vi "X Table Stage Manufacturer Model - FGV.vi"(7 "Actions":T2=enum."Clear", 8 "Error In":errorcluster, 11 "Device Type [In]":T1 caption="Device Type") -> (0 "Error Out":errorcluster, 3 "X Out":T1 caption="Device Type [Out]")   [LabVIEW 2014]
uses:
  General/Controls/FGV Actions.ctl
  General/Controls/Translation Stage Types.ctl
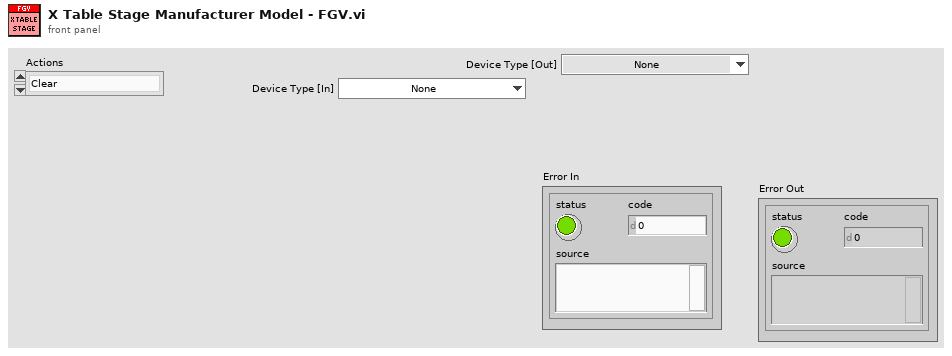
[diagram p1: front panel]
types:
  T1 = typedef "Translation Stage Types.ctl" = enum16{"None", "Thorlabs LTS", "Thorlabs MLJ"}
  T2 = typedef "FGV Actions.ctl" = enum16{"Init", "Set", "Get", "Clear"}
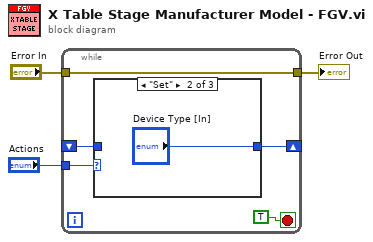
[diagram p0: block diagram]
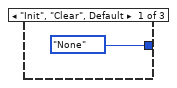
[diagram p2: hidden frame]
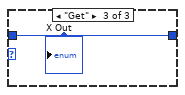
[diagram p3: hidden frame]
diagram:
  n1 = while {
    tunnel: "Actions" -> [w8]
    shift-right: [w6] -> _
    shift-left: _ -> [w5]
    tunnel: [w4] -> w2
    tunnel: "Error In" -> [w4]
    stop <- TRUE stop-if-true
    n2 = case shown="\"Set\"" w8 {
      tunnel: [Translation_Stage_Types."None" ("X") "Device Type [In]" w11] -> w6
      tunnel: w5 -> [_ _ w11]
      frame "Init", "Clear", Default {
      }
      frame "Set" {
      }
      frame "Get" {
        "X Out" <- w11
      }
    }
  }
  "Error Out" <- w2
